vi "sensitivity_.vi"(8 "error in (no error)":errorcluster, 9 "Sensitivity In":u16(ring) items=["10 uV"=11, "20 uV"=12, "50 uV"=13, "100 uV"=14, "200 uV"=15, "500 uV"=16, "1mV"=17, "2 mV"=18, "5 mV"=19, "10 mV"=20, "20 mV"=21, "50 mV"=22, "100 mV"=23, "200 mV"=24, "500 mV"=25, "1 V"=26], 11 "VISA resource name":refnum<visa-resource-name>) -> (0 "error out":errorcluster, 3 "VISA resource name out":refnum<visa-resource-name>)   [LabVIEW 2014]
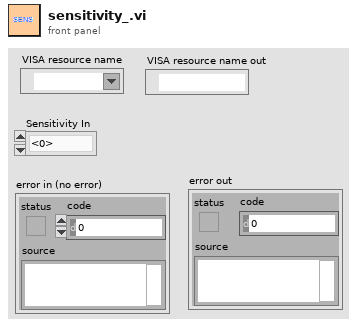
[diagram p1: front panel]
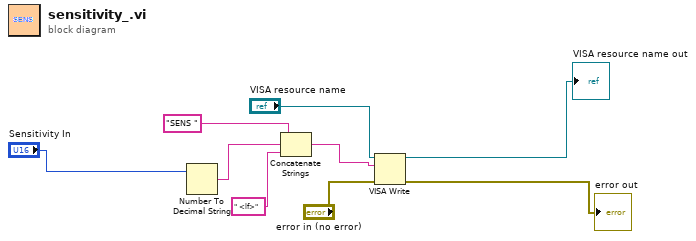
[diagram p0: block diagram]
diagram:
  n1 = Number To Decimal String(number="Sensitivity In") -> (decimal integer string=w5:string)  [unwired: 1 in]
  n2 = Concatenate Strings("SENS " ("string"), w5, " <lf>" ("string")) -> (w4:string)
  n3 = VISA Write(VISA resource name="VISA resource name", write buffer=w4, error in (no error)="error in (no error)") -> (VISA resource name out=→"VISA resource name out":refnum<visa-resource-name>, error out=→"error out":errorcluster)  [unwired: 1 out]
